vi "ROS_Publisher.vi"() -> ()   [LabVIEW 2016]
doc: "The ROS publisher bundles together several variables into a \"MasterMessage\" that is published on the ROS network. If there is an error in the ROS Write node the VI is exited."
uses:
  builds/UnicornMain/UnicornRIO1/ROS for LabVIEW/home/lvuser/natinst/bin/user.lib/ROS for LabVIEW Software/ROS/Code/SubVIs/_ROSControl.ctl
  builds/UnicornMain/UnicornRIO1/ROS for LabVIEW/home/lvuser/natinst/bin/user.lib/ROS for LabVIEW Software/ROS/Code/SubVIs/_ROSDirection.ctl
  builds/UnicornMain/UnicornRIO1/ROS for LabVIEW/home/lvuser/natinst/bin/user.lib/ROS for LabVIEW Software/ROS/Code/Console/Servers/ServerSubs/TopicDef.ctl
  builds/ROS_Test1/UnicornRIO1/ROS for LabVIEW/home/lvuser/natinst/bin/user.lib/ROS for LabVIEW Software/ROS/Code/_ROSDefinition.vi
  GlobalVI.vi
panel:
  out "msg out":string
  out "Array":dbl[](array[numeric])
  out "PickingRoutine":i32
  out "ROS out":T1={"topic port"=0, "Node"="", "topic"="", "type"="", "node port"=0, "error "={"status"=FALSE, "code"=0, "source"=""}, "Direction"=enum."Node", "Update (ms)"=1, "FIFO size"=1}
  out "position":cluster{"x":dbl, "y":dbl, "z":dbl}
  out "ROS Write ERR":errorcluster
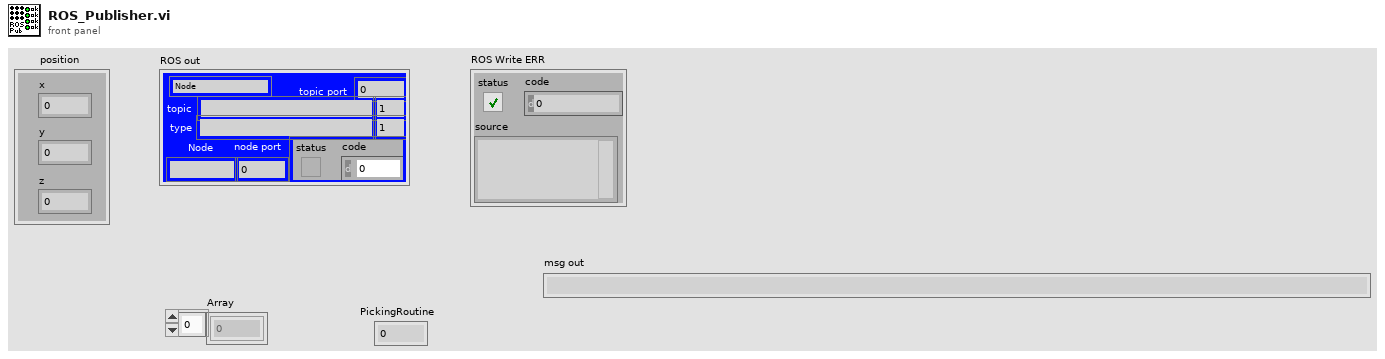
[diagram p1: front panel]
types:
  T1 = typedef "_ROSControl.ctl" = cluster{"topic port":u16, "Node":string, "topic":string, "type":string, "node port":u16, "error ":errorcluster, "Direction":T2, "Update (ms)":u16, "FIFO size":u16}
  T2 = typedef "_ROSDirection.ctl" = enum16{"Node", "Publisher", "Subscriber", "ServiceClient", "ServiceProvider"}
  T3 = typedef "TopicDef.ctl" = cluster{"Topic":string, "Type":string, "Action":T2, "Update (ms)":u16, "queue size":u16}
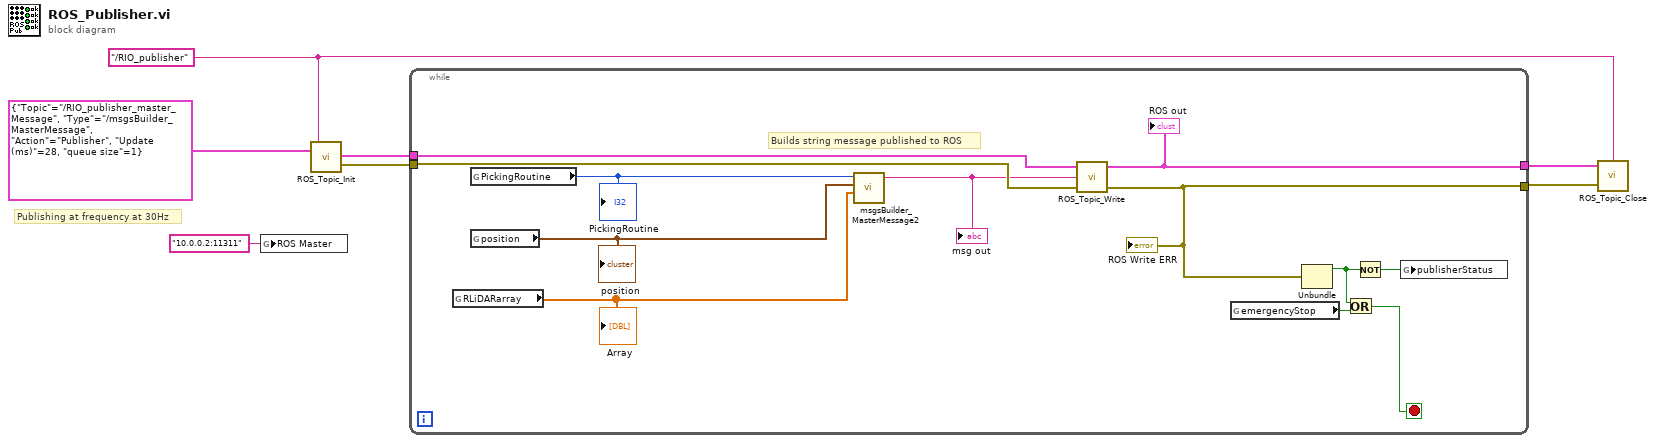
[diagram p0: block diagram]
diagram:
  w2 = "/RIO_publisher" ("node")
  # "Publishing at frequency at 30Hz"
  n1 = global write "_ROSDefinition.vi" "ROS Master"("10.0.0.2:11311" ("ROS Master")) -> ()
  n2 = call "ROS_Topic_Init.vi"("Definitions"=T3 {"Topic"="/RIO_publisher_master_Message", "Type"="/msgsBuilder_MasterMessage", "Action"=enum."Publisher", "Update (ms)"=28, "queue size"=1}, "node"=w2) -> ("ROS out"=w4:T1, "error out"=w1:errorcluster)  [unwired: 1 in]
  n3 = while {
    tunnel: [w16] -> w6
    tunnel: [w15] -> w5
    tunnel: w4 -> [w14]
    tunnel: w1 -> [w13]
    stop <- w12 stop-if-true
    # "Builds string message published to ROS"
    n4 = global read "GlobalVI.vi" "RLiDARarray"() -> (w8:dbl[])
    "Array" <- w8
    n5 = global read "GlobalVI.vi" "PickingRoutine"() -> (w9:i32)
    "PickingRoutine" <- w9
    n6 = global read "GlobalVI.vi" "position"() -> (w10:cluster{"x":dbl, "y":dbl, "z":dbl})
    "position" <- w10
    n7 = call "msgsBuilder_MasterMessage2.vi"("Array"=w8, "position in"=w10, "liftState"=w9) -> ("msg out"=w11:string)  [unwired: 8 in]
    "msg out" <- w11
    n8 = call "ROS_Topic_Write.vi"("error in (no error)"=w13, "Msg in"=w11, "ROS in"=w14) -> ("error out"=w15:errorcluster, "ROS out"=w16:T1)  [unwired: 1 in]
    "ROS Write ERR" <- w15
    "ROS out" <- w16
    n9 = global read "GlobalVI.vi" "emergencyStop"() -> (w19:bool)
    n10 = Unbundle(w15) -> ("status"=w17:bool)  [unwired: 2 out]
    n11 = Or(x=w17, y=w19) -> (x .or. y?=w12:bool)
    n12 = Not(x=w17) -> (.not. x?=w18:bool)
    n13 = global write "GlobalVI.vi" "publisherStatus"(w18) -> ()
  }
  n14 = call "ROS_Topic_Close.vi"("error in"=w5, "ROS in"=w6, "node"=w2) -> ()  [unwired: 1 in, 1 out]
